vi "Send Toggle Output.vi"(8 "error in":errorcluster, 11 "69X_79X in":refnum<class "7976A.lvclass">) -> (0 "error out":errorcluster, 3 "69X_79X out":refnum<class "7976A.lvclass">)   [LabVIEW 2019, in "7976A.lvlib" / "7976A.lvclass"]
uses:
  Library/7976A.lvclass
  C:/Users/Public/Documents/Development/builds/Instruments/PowerSupply.lvlibp/Library/PowerSupply.lvclass
  Accessors/Read Local Resource.vi
  Accessors/Write Local Resource.vi
  <instrlib>/Agilent N7976A/Agilent N7976A.lvlib
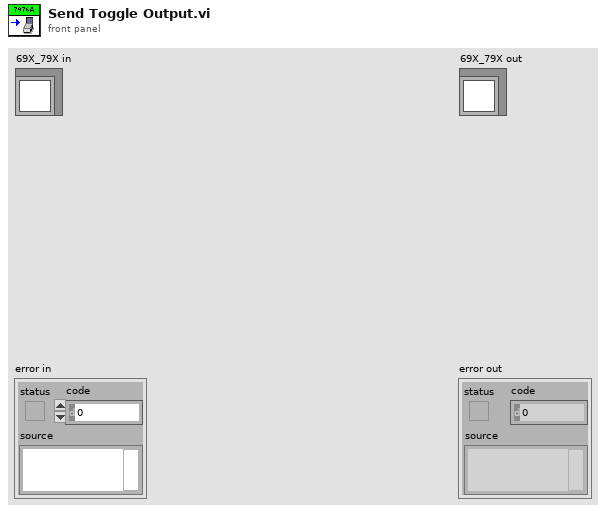
[diagram p1: front panel]
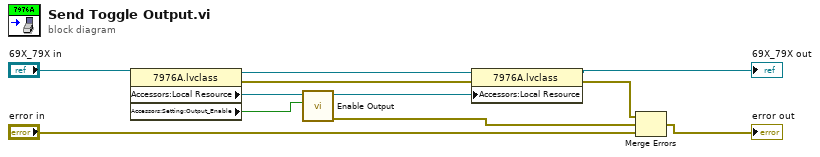
[diagram p0: block diagram]
diagram:
  n1 = property class="7976A.lvclass"(reference="69X_79X in") -> (reference out=w10:refnum<class "7976A.lvclass">, error out=w9:errorcluster, "Accessors:Local Resource"=w4:refnum<visa-resource-name>, "Accessors:Setting:Output_Enable"=w1:bool)  [unwired: 1 in]
  n2 = call <instrlib>:"Enable Output.vi"("Enable Output (F: Disable)"=w1, "VISA resource name"=w4) -> ("error out"=w2:errorcluster, "VISA resource name out"=w3:refnum<visa-resource-name>)  [unwired: 8 in]
  n3 = property class="7976A.lvclass"(reference=w10, error in=w9, "Accessors:Local Resource"=w3) -> (reference out=→"69X_79X out":refnum<class "7976A.lvclass">, error out=w7:errorcluster)
  n4 = Merge Errors(w7, w2, "error in") -> (→"error out":errorcluster)
